vi "获取绝对路径.vi"(1 "relativePath":string) -> (0 "absolutePath":path)   [LabVIEW 2014]
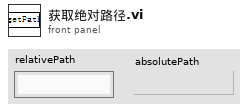
[diagram p1: front panel]
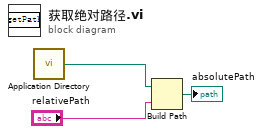
[diagram p0: block diagram]
diagram:
  n1 = call <vilib>:"Application Directory.vi"() -> ("Application Directory"=w3:path)
  n2 = Build Path(base path=w3, name or relative path="relativePath") -> (appended path=→"absolutePath":path)
